vi "Picture to 2-D Color Array.vi"(8 "error in":errorcluster, 10 "input cluster":cluster{"Width":u32, "Height":u32}, 11 "picture":picture) -> (0 "error out":errorcluster, 3 "Color Array":cluster{"Red":u8, "Green":u8, "Blue":u8}[][](array[cluster]))   [LabVIEW 2019, in "Initializers.lvlib"]
uses:
  Initializers.lvlib
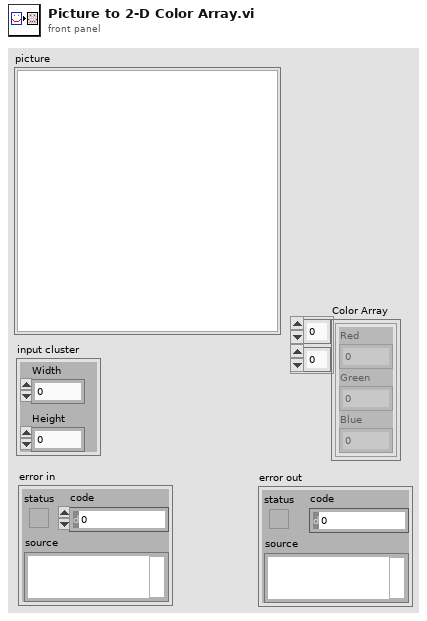
[diagram p1: front panel]
types:
  T1 = cluster{"left":i16, "top":i16, "right":i16, "bottom":i16}
  T2 = typedef "imagedata.ctl" = cluster{"image type":i32, "image depth":i32, "image":u8[], "mask":u8[], "colors":u32[], "Rectangle":cluster{"left":i16, "top":i16, "right":i16, "bottom":i16}}
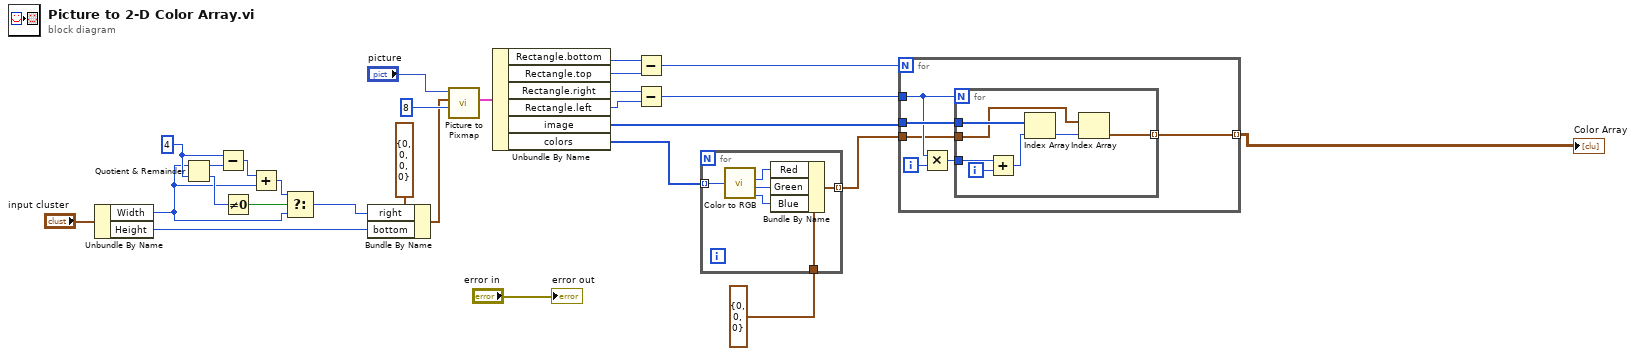
[diagram p0: block diagram]
diagram:
  w12 = 4
  n1 = Unbundle By Name("input cluster") -> ("Width"=w5:u32, "Height"=w16:u32)
  n2 = Quotient & Remainder(x=w5, y=w12) -> (x-y*floor(x/y)=w11:u32, floor(x/y)=w10:u32)
  n3 = Subtract(x=w12, y=w11) -> (x-y=w4:u32)
  n4 = Not Equal To 0?(x=w10) -> (x != 0?=w9:bool)
  n5 = Add(x=w4, y=w5) -> (x+y=w3:u32)
  n6 = Select(t=w3, s=w9, f=w5) -> (s? t:f=w2:u32)
  n7 = Bundle By Name(cluster=T1 {"left"=0, "top"=0, "right"=0, "bottom"=0} ("rect"), "right"=w2, "bottom"=w16) -> (w13:T1)
  n8 = call <vilib>:"Picture to Pixmap.vi"("depth"=8, "rect"=w13, "picture"="picture") -> ("image data"=w17:T2)  [unwired: 7 in, 1 out]
  n9 = Unbundle By Name(w17) -> ("Rectangle.bottom"=w20:i16, "Rectangle.top"=w21:i16, "Rectangle.right"=w23:i16, "Rectangle.left"=w24:i16, "image"=w26:u8[], "colors"=w8:u32[])
  n10 = Subtract(x=w20, y=w21) -> (x-y=w22:i16)
  n11 = Subtract(x=w23, y=w24) -> (x-y=w25:i16)
  n12 = for {
    tunnel: w8 -> [w33] mode=indexing
    tunnel: cluster{"Red":u8, "Green":u8, "Blue":u8} {"Red"=0, "Green"=0, "Blue"=0} ("Cluster") -> [w32]
    tunnel: [w28] -> w6 mode=indexing
    n13 = call <vilib>:"Color to RGB.vi"("Color"=w33) -> ("R"=w30:u8, "G"=w31:u8, "B"=w29:u8)  [unwired: 1 out]
    n14 = Bundle By Name(cluster=w32, "Red"=w30, "Green"=w31, "Blue"=w29) -> (w28:cluster{"Red":u8, "Green":u8, "Blue":u8})
  }
  n15 = for {
    N: w22 -> [_]
    tunnel: w6 -> [w36]
    tunnel: w25 -> [w37]
    tunnel: w26 -> [w39]
    tunnel: [w34] -> w1 mode=indexing
    i -> [w38]
    n16 = Multiply(x=w37, y=w38) -> (x*y=w35:i32)
    n17 = for {
      N: w37 -> [_]
      tunnel: w39 -> [w46]
      tunnel: w36 -> [w41]
      tunnel: w35 -> [w45]
      tunnel: [w40] -> w34 mode=indexing
      i -> [w44]
      n18 = Add(x=w45, y=w44) -> (x+y=w43:i32)
      n19 = Index Array(array=w46, index=w43) -> (element=w42:u8)
      n20 = Index Array(array=w41, index=w42) -> (element=w40:cluster{"Red":u8, "Green":u8, "Blue":u8})
    }
  }
  "Color Array" <- w1
  "error out" <- "error in"
